vi "rvc Rotate Matrix.vi"(6 "angle unit":u16(ring)=1 items=["degree", "radians"], 9 "vector":dbl[](array[numeric])=[1.0, 0.0, 0.0], 10 "angle":dbl, 11 "rotation matrix in":T1) -> (3 "rotation matrix":T1)   [LabVIEW 2017]
uses:
  <vilib>/Analysis/Matrix/Datatypes/RealMatrix.ctl
  <vilib>/Analysis/baseanly.llb/Real A x B.vi
  <vilib>/Analysis/_algsub.llb/Vector Norm.vi
  <vilib>/Analysis/_algsub.llb/Real Vector Norm.vi
  <vilib>/Analysis/baseanly.llb/Outer Product.vi
  <vilib>/Analysis/baseanly.llb/Real Outer Product.vi
  <vilib>/robotics/Kinematics/Create Lie Group Matrix.vi
  <vilib>/Analysis/7linalg.llb/Create Special Matrix.vi
  <vilib>/Analysis/7linalg.llb/Create Special Real Matrix.vi
  <vilib>/Analysis/Matrix/Numeric/Multiply/Multiply.vi
  <vilib>/Analysis/Matrix/Numeric/Multiply/Multiply - RM,R.vi
  <vilib>/Analysis/Matrix/Numeric/Multiply/Multiply - R,RM.vi
  <vilib>/Analysis/Matrix/Numeric/Add/Add.vi
  <vilib>/Analysis/Matrix/Numeric/Add/Add - RM,RM.vi
  <vilib>/robotics/Kinematics/NI_Kinematics.lvlib
  <vilib>/Analysis/NI_AALBase.lvlib
  <vilib>/Analysis/Matrix/NI_Matrix.lvlib
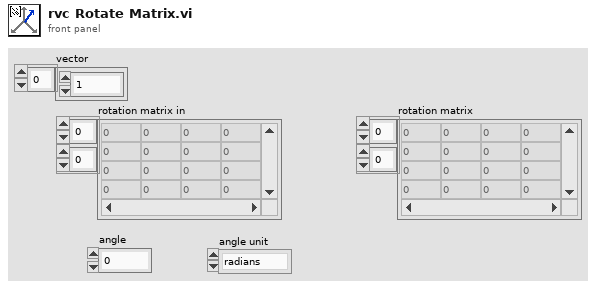
[diagram p1: front panel]
types:
  T1 = typedef "NI_Matrix.lvlib/RealMatrix.ctl" = dbl[][]
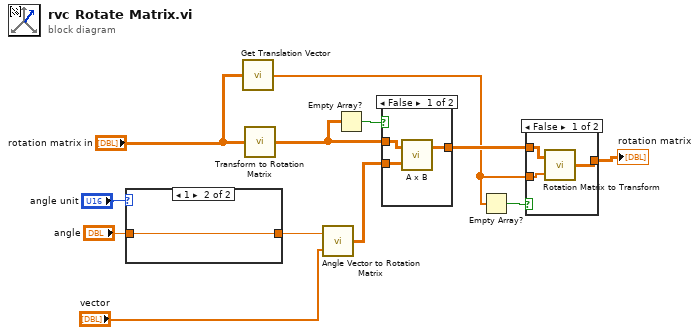
[diagram p0: block diagram]
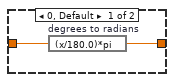
[diagram p3: hidden frame]
diagram:
  n1 = case shown="1" "angle unit" {
    tunnel: "angle" -> [w14 w15]
    tunnel: [w13 w15] -> w7
    frame 0, Default {
      n2 = expression code="(x/180.0)*pi" "degrees to radians"(w14) -> (w13:dbl)
    }
    frame 1 {
    }
  }
  n3 = call <vilib>:"Get Translation Vector.vi"("transform"="rotation matrix in") -> ("translation vector"=w2:dbl[])
  n4 = call <vilib>:"Transform to Rotation Matrix.vi"("transform"="rotation matrix in") -> ("rotation matrix"=w6:T1)
  n5 = call <vilib>:"Angle Vector to Rotation Matrix.vi"("vector"="vector", "angle"=w7) -> ("rotation matrix"=w11:T1)
  n6 = Empty Array?(array=w6) -> (empty?=w10:bool)
  n7 = case shown="False" w10 {
    tunnel: w11 -> [w18 w19]
    tunnel: w6 -> [w17 _]
    tunnel: [w16 w19] -> w4
    frame False {
      n8 = call-poly <vilib>:"A x B.vi"("B"=w18, "A"=w17) -> ("A x B"=w16:T1)  [unwired: 1 out]
    }
    frame True {
    }
  }
  n9 = Empty Array?(array=w2) -> (empty?=w1:bool)
  n10 = case shown="False" w1 {
    tunnel: w4 -> [w22 w23]
    tunnel: [w21 w23] -> w3
    tunnel: w2 -> [w20 _]
    frame False {
      n11 = call <vilib>:"Rotation Matrix to Transform.vi"("translation vector"=w20, "rotation matrix"=w22) -> ("transform"=w21:T1)
    }
    frame True {
    }
  }
  "rotation matrix" <- w3
